vi "LogStringEvent(Caller).vi"(8 "Error In":errorcluster, 10 "Data":string, 11 "Field":string) -> (0 "Error Out":errorcluster)   [LabVIEW 2019, in "EventLogger.lvlib"]
uses:
  EventLogger.lvlib
  Enum - Message.ctl
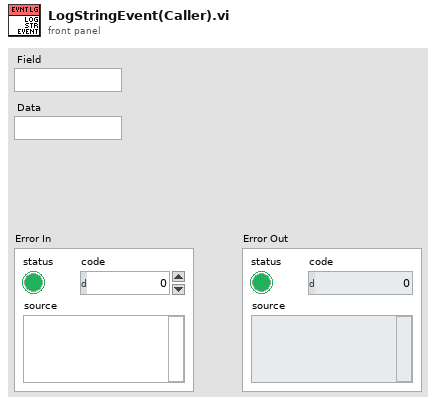
[diagram p1: front panel]
types:
  T1 = typedef "EventLogger.lvlib/Enum - Message.ctl" = enum16{"Initialize", "Idle", "CreateLog", "LogStrEvent", "LogErrorEvent", "LogVICall", "Error", "Exit"}
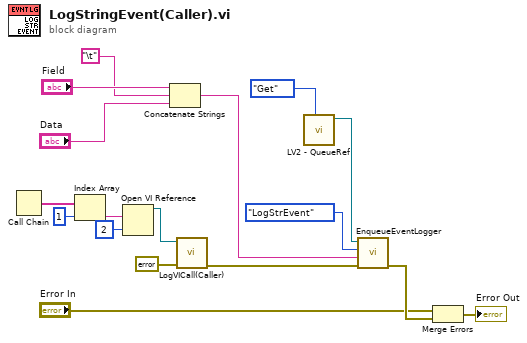
[diagram p0: block diagram]
diagram:
  n1 = Call Chain() -> (call chain=w8:string[])
  n2 = Index Array(array=w8, index=1) -> (element=w6:string)
  n3 = Open VI Reference(vi path=w6, options=2) -> (vi reference=w4:refnum<vi>)  [unwired: 4 in, 1 out]
  n4 = Concatenate Strings("Field", "\t", "Data") -> (w10:string)
  n5 = call "LogVICall(Caller).vi"("Error In"=errorcluster {"status"=FALSE, "code"=0, "source"=""}, "Caller VI"=w4) -> ("Error Out"=w9:errorcluster)  [unwired: 9 in]
  n6 = call "LV2 - QueueRef.vi"("Action"=enum16{"Set", "Get"}."Get") -> ("EventLoggerQueue out"=w15:refnum<queue>)  [unwired: 10 in]
  n7 = call "EnqueueEventLogger.vi"("Error In"=w9, "Data"=w10, "Message"=Enum_-_Message."LogStrEvent", "EventLoggerQueue"=w15) -> ("Error Out"=w16:errorcluster)  [unwired: 6 in, 1 out]
  n8 = Merge Errors("Error In", w16) -> (→"Error Out":errorcluster)
